vi "p1.vi"() -> ()   [LabVIEW 2021, in "d10.lvlib"]
uses:
  d10.lvlib
  AOC/AOC.lvlib
panel:
  in  "Example":string="addx 15\naddx -11\naddx 6\naddx -3\naddx 5\naddx -1\naddx -8\naddx 13\naddx 4\nnoop\naddx -1\naddx 5\naddx -1\naddx 5\naddx -1\naddx 5\naddx -1\naddx 5\naddx -1\naddx -35\naddx 1\naddx 24\naddx -19\naddx 1\naddx 16\naddx -11\nnoop\nnoop\naddx 21\naddx -15\nnoop\nnoop\naddx -3\naddx 9\naddx 1\naddx -3\naddx 8\naddx 1\naddx 5\nnoop\nnoop\nnoop\nnoop\nnoop\naddx -36\nnoop\naddx 1\naddx 7\nnoop\nnoop\nnoop\naddx 2\naddx 6\nnoop\nnoop\nnoop\nnoop\nnoop\naddx 1\nnoop\nnoop\naddx 7\naddx 1\nnoop\naddx -13\naddx 13\naddx 7\nnoop\naddx 1\naddx -33\nnoop\nnoop\nnoop\naddx 2\nnoop\nnoop\nnoop\naddx 8\nnoop\naddx -1\naddx 2\naddx 1\nnoop\naddx 17\naddx -9\naddx 1\naddx 1\naddx -3\naddx 11\nnoop\nnoop\naddx 1\nnoop\naddx 1\nnoop\nnoop\naddx -13\naddx -19\naddx 1\naddx 3\naddx 26\naddx -30\naddx 12\naddx -1\naddx 3\naddx 1\nnoop\nnoop\nnoop\naddx -9\naddx 18\naddx 1\naddx 2\nnoop\nnoop\naddx 9\nnoop\nnoop\nnoop\naddx -1\naddx 2\naddx -37\naddx 1\naddx 3\nnoop\naddx 15\naddx -21\naddx 22\naddx -6\naddx 1\nnoop\naddx 2\naddx 1\nnoop\naddx -10\nnoop\nnoop\naddx 20\naddx 1\naddx 2\naddx 2\naddx -6\naddx -11\nnoop\nnoop\nnoop"
  in  "Example":bool
  out "Answer":i64=11960
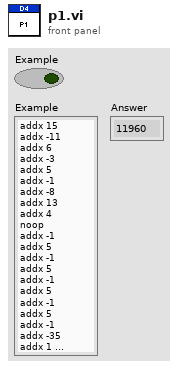
[diagram p1: front panel]
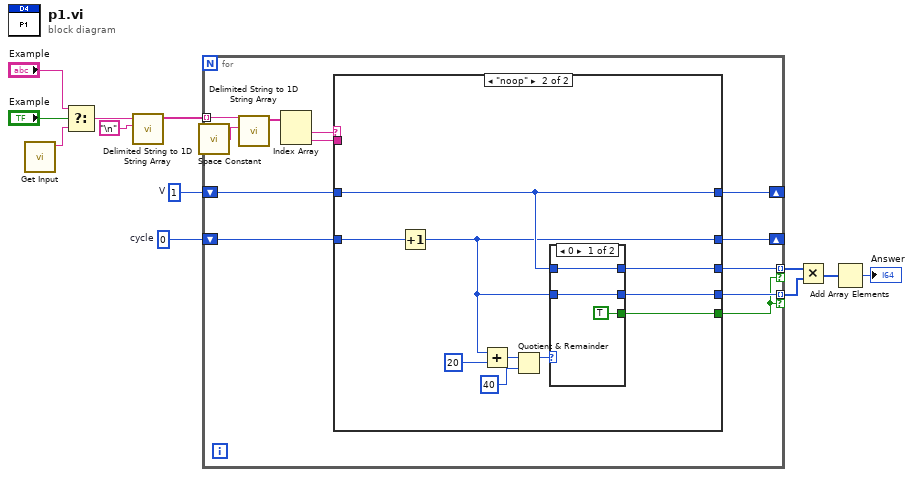
[diagram p0: block diagram]
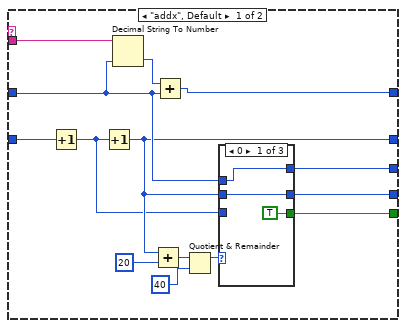
[diagram p2: hidden frame]
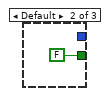
[diagram p3: hidden frame]
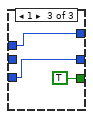
[diagram p4: hidden frame]
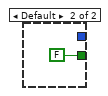
[diagram p5: hidden frame]
diagram:
  w5 = i64 0  # cycle
  w6 = i64 1  # V
  n1 = call "Get Input.vi"() -> ("Input"=w12:string)  [unwired: 11 in]
  n2 = Select(t="Example", s="Example", f=w12) -> (s? t:f=w11:string)
  n3 = call <vilib>:"Delimited String to 1D String Array.vi"("delimiter"="\n", "delimited string"=w11) -> ("string array"=w7:string[])  [unwired: 9 in]
  n4 = for {
    tunnel: w7 -> [w24] mode=indexing
    shift-right: [w18] -> _
    shift-left: w6 -> [w20]
    shift-right: [w17] -> _
    shift-left: w5 -> [w19]
    tunnel: [w15] -> w3 mode=indexing if=w13
    tunnel: [w14] -> w4 mode=indexing if=w13
    n5 = call <vilib>:"Space Constant.vi"() -> ("String"=w23:string)
    n6 = call <vilib>:"Delimited String to 1D String Array.vi"("delimiter"=w23, "delimited string"=w24) -> ("string array"=w22:string[])  [unwired: 9 in]
    n7 = Index Array(array=w22) -> (element #1=w21:string, element #2=w16:string)  [unwired: 2 in]
    n8 = case shown="\"noop\"" w21 {
      tunnel: w20 -> [w34 w52]
      tunnel: w19 -> [w29 w51]
      tunnel: [w33 w52] -> w18
      tunnel: [w30 w46] -> w17
      tunnel: w16 -> [w38 _]
      tunnel: [w32 w55] -> w15
      tunnel: [w31 w54] -> w14
      tunnel: [w28 w53] -> w13
      frame "addx", Default {
        n9 = Increment(x=w29) -> (x+1=w27:i64)
        n10 = Increment(x=w27) -> (x+1=w30:i64)
        n11 = Decimal String To Number(string=w38, default (0L)=w34) -> (number=w37:i64)  [unwired: 1 in, 1 out]
        n12 = Add(x=w30, y=i64 20 ("x")) -> (x+y=w26:i64)
        n13 = Add(x=w37, y=w34) -> (x+y=w33:i64)
        n14 = Quotient & Remainder(x=w26, y=i64 40) -> (x-y*floor(x/y)=w35:i64)  [unwired: 1 out]
        n15 = case shown="0" w35 {
          tunnel: w30 -> [w41 _ _]
          tunnel: w34 -> [w39 _ w44]
          tunnel: [w39 _ w44] -> w32
          tunnel: [w41 _ w43] -> w31
          tunnel: [TRUE FALSE TRUE] -> w28
          tunnel: w27 -> [_ _ w43]
          frame 0 {
          }
          frame Default {
          }
          frame 1 {
          }
        }
      }
      frame "noop" {
        n16 = Increment(x=w51) -> (x+1=w46:i64)
        n17 = Add(x=w46, y=i64 20 ("x")) -> (x+y=w49:i64)
        n18 = Quotient & Remainder(x=w49, y=i64 40) -> (x-y*floor(x/y)=w47:i64)  [unwired: 1 out]
        n19 = case shown="0" w47 {
          tunnel: w46 -> [w58 _]
          tunnel: [w57 _] -> w55
          tunnel: w52 -> [w57 _]
          tunnel: [w58 _] -> w54
          tunnel: [TRUE FALSE] -> w53
          frame 0 {
          }
          frame Default {
          }
        }
      }
    }
  }
  n20 = Multiply(x=w3, y=w4) -> (x*y=w2:i64[])
  n21 = Add Array Elements(numeric array=w2) -> (sum=→"Answer":i64)
